vi "svl_Max-Min Level with IC.vi"(6 "initial min level":dbl format="%.2f", 7 "initial max level":dbl format="%.2f", 8 "error in (no error)":errorcluster, 9 "processing state":T1(ring), 11 "scaled signal":waveform(dbl)={"t0"=timestamp(0 s since 1904-01-01), "dt"=0.0, "Y"=[]}) -> (0 "error out":errorcluster, 2 "max-min level":dbl format="%.2f", 4 "final min level":dbl format="%.2f", 5 "final max level":dbl format="%.2f")   [LabVIEW 2017]
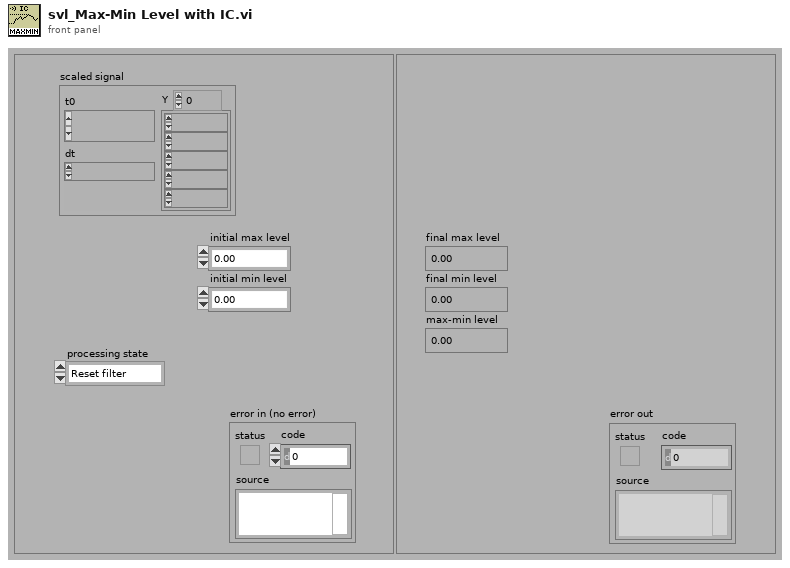
[diagram p1: front panel]
types:
  T1 = enum16{"Reset filter", "Restart averaging", "Continue processing"}
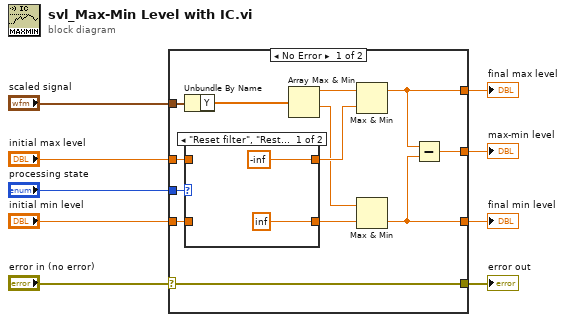
[diagram p0: block diagram]
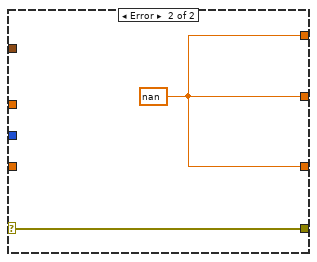
[diagram p3: hidden frame]
diagram:
  n1 = case shown="No Error" "error in (no error)" {
    selector: "error in (no error)" -> [w22 w28]
    tunnel: [w22 w28] -> w7
    tunnel: "scaled signal" -> [w20 _]
    tunnel: "processing state" -> [w21 _]
    tunnel: "initial max level" -> [w17 _]
    tunnel: [w13 w27] -> w9
    tunnel: "initial min level" -> [w18 _]
    tunnel: [w12 w27] -> w2
    tunnel: [w11 w27] -> w1
    frame No Error {
      n2 = Unbundle By Name(w20) -> ("Y"=w10:dbl[])
      n3 = case shown="\"Reset filter\", \"Restart averaging\", Default" w21 {
        tunnel: w17 -> [_ w26]
        tunnel: [-inf ("t") w26] -> w16
        tunnel: w18 -> [_ w25]
        tunnel: [inf ("t") w25] -> w14
        frame "Reset filter", "Restart averaging", Default {
        }
        frame "Continue processing" {
        }
      }
      n4 = Array Max & Min(array=w10) -> (max value=w19:dbl, min value=w15:dbl)  [unwired: 2 out]
      n5 = Max & Min(x=w19, y=w16) -> (max(x,y)=w13:dbl)  [unwired: 1 out]
      n6 = Max & Min(x=w15, y=w14) -> (min(x,y)=w12:dbl)  [unwired: 1 out]
      n7 = Subtract(x=w13, y=w12) -> (x-y=w11:dbl)
    }
    frame Error {
      w27 = nan ("soundLevel")
    }
  }
  "final max level" <- w9
  "error out" <- w7
  "final min level" <- w2
  "max-min level" <- w1
